vi "Insert SubPanel.vi"(8 "error in (no error)":errorcluster, 10 "VI Ref":refnum<vi>, 11 "Subpanel Ref":refnum<vi>) -> (0 "error out":errorcluster)   [LabVIEW 2019]
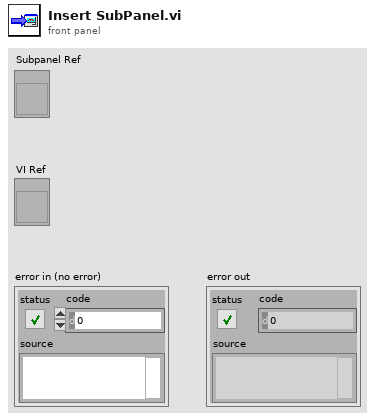
[diagram p1: front panel]
types:
  T1 = enum32{"Invalid", "Standard", "Closed", "Hidden", "Minimized", "Maximized"}
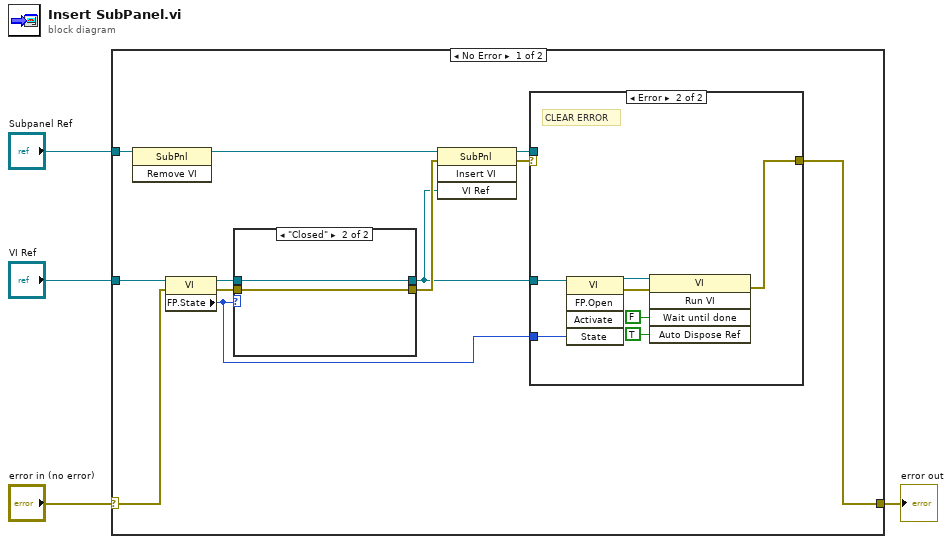
[diagram p0: block diagram]
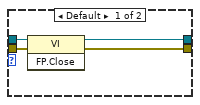
[diagram p2: hidden frame]
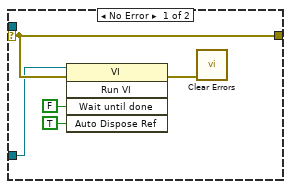
[diagram p3: hidden frame]
diagram:
  n1 = case shown="No Error" "error in (no error)" {
    selector: "error in (no error)" -> [w8 w35]
    tunnel: "VI Ref" -> [w16 _]
    tunnel: "Subpanel Ref" -> [w6 _]
    tunnel: [w7 w35] -> w1
    frame No Error {
      n2 = invoke class="SubPnl" method="Remove VI"(reference=w6) -> (reference out=w5:refnum<vi>)  [unwired: 2 in, 2 out]
      n3 = property class="VI"(reference=w16, error in=w8) -> (reference out=w15:refnum<vi>, error out=w14:errorcluster, "FP.State"=w9:T1)
      n4 = case shown="\"Closed\"" w9 {
        tunnel: w15 -> [w20 w21]
        tunnel: w14 -> [w19 w22]
        tunnel: [w18 w21] -> w10
        tunnel: [w17 w22] -> w13
        frame Default {
          n5 = invoke class="VI" method="FP.Close"(reference=w20, error in=w19) -> (reference out=w18:refnum<vi>, error out=w17:errorcluster)  [unwired: 1 in, 1 out]
        }
        frame "Closed" {
        }
      }
      n6 = invoke class="SubPnl" method="Insert VI"(reference=w5, error in=w13, "VI Ref"=w10) -> (reference out=w11:refnum<vi>, error out=w12:errorcluster)  [unwired: 1 in, 2 out]
      n7 = case shown="Error" w12 {
        selector: w12 -> [w27 _]
        tunnel: w11 -> [_ _]
        tunnel: w10 -> [w26 w34]
        tunnel: w9 -> [_ w33]
        tunnel: [w27 w30] -> w7
        frame No Error {
          n8 = invoke class="VI" method="Run VI"(reference=w26, error in=w27, "Wait until done"=FALSE ("Wait Until Done"), "Auto Dispose Ref"=TRUE ("Auto Dispose Reference")) -> (error out=w23:errorcluster)  [unwired: 1 in, 4 out]
          n9 = call <vilib>:"Clear Errors.vi"("error in (no error)"=w23) -> ()  [unwired: 5 in, 2 out]
        }
        frame Error {
          # "CLEAR ERROR"
          n10 = invoke class="VI" method="FP.Open"(reference=w34, "State"=w33) -> (reference out=w31:refnum<vi>, error out=w32:errorcluster)  [unwired: 3 in, 3 out]
          n11 = invoke class="VI" method="Run VI"(reference=w31, error in=w32, "Wait until done"=FALSE ("Wait Until Done"), "Auto Dispose Ref"=TRUE ("Auto Dispose Reference")) -> (error out=w30:errorcluster)  [unwired: 1 in, 4 out]
        }
      }
    }
    frame Error {
    }
  }
  "error out" <- w1
